vi "IMAQ FPGA Camera Link Pixel Packer U16x4.vi"(8 "Input Valid":bool, 9 "Frame Valid In":bool, 10 "Line Valid In":bool, 11 "Pixels In":u16[](array[numeric])=[0, 0, 0, 0]) -> (0 "Output Valid":bool, 1 "Frame Valid Out":bool, 2 "Line Valid Out":bool, 3 "Pixel Bus x8 Out":cluster{"Pixels":u16[], "DV":bool[]})   [LabVIEW 2020]
doc: "The Pixel Packer combines pixels from different cycles to create a Pixel Bus with 8 adjacent pixels. The DV flag in the Pixel Bus x8 Out indicates if the corresponding pixel is valid in case there are cameras with a width that is not a multiple of 8."
uses:
  <vilib>/visionFPGA/Basics/Camera Link Acquisition/Controls/IMAQ FPGA Camera Link Pixel Packer State.ctl
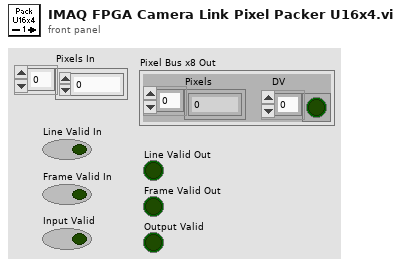
[diagram p1: front panel]
types:
  T1 = typedef "IMAQ FPGA Camera Link Pixel Packer State.ctl" = enum16{"Wait to Pack", "Pack", "Add EOL", "Check EOI"}
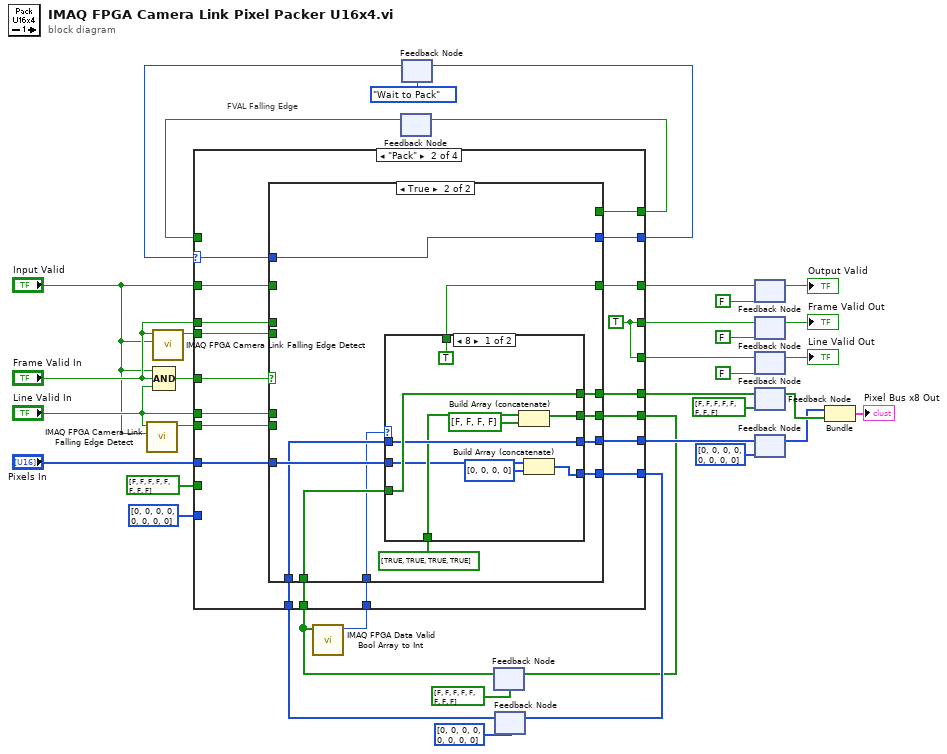
[diagram p0: block diagram]
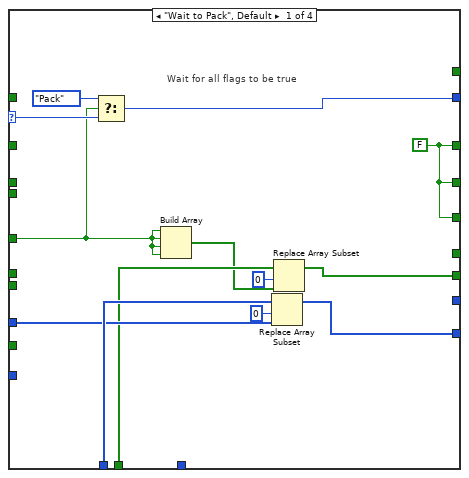
[diagram p2: hidden frame]
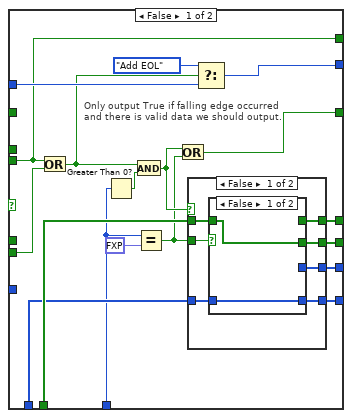
[diagram p3: hidden frame]
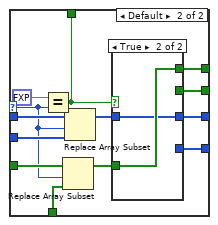
[diagram p6: hidden frame]
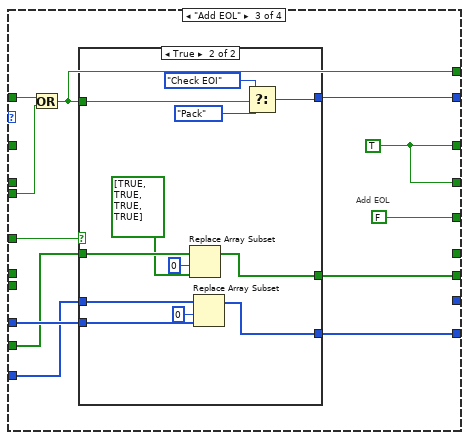
[diagram p8: hidden frame]
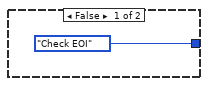
[diagram p9: hidden frame]
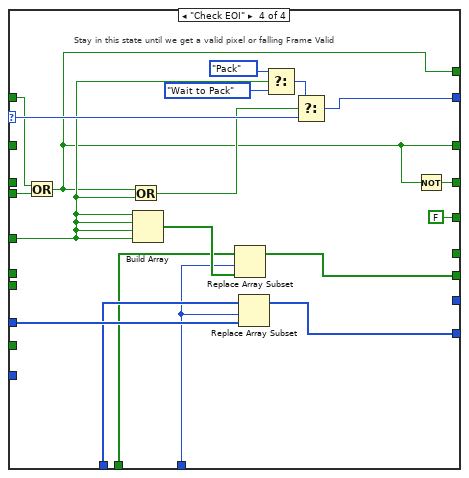
[diagram p10: hidden frame]
diagram:
  # "FVAL Falling Edge"
  n1 = call <vilib>:"IMAQ FPGA Camera Link Falling Edge Detect.vi"("Input Valid"="Input Valid", "Input"="Line Valid In") -> ("Falling Edge"=w7:bool)  [unwired: 9 in]
  n2 = call <vilib>:"IMAQ FPGA Camera Link Falling Edge Detect.vi"("Input Valid"="Input Valid", "Input"="Frame Valid In") -> ("Falling Edge"=w10:bool)  [unwired: 9 in]
  n3 = Compound Arithmetic op=AND("Input Valid", "Frame Valid In", "Line Valid In") -> (w16:bool)
  n4 = feedback #1() -> (w3:bool)  [unwired: 1 in]
  n5 = feedback #2(IMAQ_FPGA_Camera_Link_Pixel_Packer_State."Wait to Pack" ("Enum")) -> (w18:T1)
  n6 = feedback #3(bool[] [FALSE, FALSE, FALSE, FALSE, FALSE, FALSE, FALSE, FALSE]) -> (w2:bool[])
  n7 = call <vilib>:"IMAQ FPGA Data Valid Bool Array to Int.vi"("DV In"=w2) -> ("Sum DV Out"=w1:u8)  [unwired: 10 in]
  n8 = feedback #4(u16[] [0, 0, 0, 0, 0, 0, 0, 0] ("Pixels")) -> (w30:u16[])
  n9 = case shown="\"Pack\"" w18 {
    selector: w18 -> [w50 w68 _ w181]
    tunnel: w2 -> [w44 w56 _ w163]
    tunnel: w30 -> [w48 w67 _ w165]
    tunnel: [_ w64 _ _] -> w29
    tunnel: [_ w63 _ _] -> w22
    tunnel: [w38 w62 w149 w166] -> w36
    tunnel: [w38 w53 w149 w168] -> w20
    tunnel: [w38 w53 FALSE FALSE ("Frame Valid In")] -> w19
    tunnel: "Frame Valid In" -> [_ w60 _ _]
    tunnel: "Line Valid In" -> [_ w61 _ _]
    tunnel: "Input Valid" -> [_ w59 _ _]
    tunnel: w16 -> [w40 w69 w148 w172]
    tunnel: "Pixels In" -> [w46 w57 w145 w176]
    tunnel: [w45 w66 w144 w174] -> w14
    tunnel: [w42 w65 w146 w175] -> w13
    tunnel: [w41 w58 w147 w180] -> w12
    tunnel: w10 -> [_ w55 w140 w170]
    tunnel: w7 -> [_ w54 _ _]
    tunnel: u16[] [0, 0, 0, 0, 0, 0, 0, 0] ("Pixels") -> [_ _ w142 _]
    tunnel: bool[] [FALSE, FALSE, FALSE, FALSE, FALSE, FALSE, FALSE, FALSE] -> [_ _ w141 _]
    tunnel: [_ w52 w138 w166] -> w4
    tunnel: w3 -> [_ _ w139 w169]
    tunnel: w1 -> [_ w51 _ w164]
    frame "Wait to Pack", Default {
      w38 = FALSE
      # "Wait for all flags to be true"
      n10 = Select(t=IMAQ_FPGA_Camera_Link_Pixel_Packer_State."Pack", s=w40, f=w50) -> (s? t:f=w41:T1)
      n11 = Build Array(w40, w40, w40, w40) -> (w39:bool[])
      n12 = Replace Array Subset(array=w48, new element=w46, index=0) -> (w45:u16[])
      n13 = Replace Array Subset(array=w44, new element=w39, index=0) -> (w42:bool[])
    }
    frame "Pack" {
      w53 = TRUE ("Frame Valid In")
      n14 = case shown="True" w69 {
        tunnel: w68 -> [w86 w110]
        tunnel: [w84 w110] -> w58
        tunnel: w67 -> [w80 w105]
        tunnel: [w76 w103] -> w66
        tunnel: w56 -> [w81 w111]
        tunnel: [w77 w107] -> w65
        tunnel: [w78 w104] -> w64
        tunnel: [w79 w108] -> w63
        tunnel: w59 -> [_ _]
        tunnel: [w70 w109] -> w62
        tunnel: w60 -> [_ _]
        tunnel: w61 -> [_ _]
        tunnel: w55 -> [w75 _]
        tunnel: w54 -> [w87 _]
        tunnel: w51 -> [w74 w101]
        tunnel: w57 -> [_ w106]
        tunnel: [w75 _] -> w52
        frame False {
          # "Only output True if falling edge occurred and there is valid data we should output."
          n15 = Or(x=w75, y=w87) -> (x .or. y?=w82:bool)
          n16 = Greater Than 0?(x=w74) -> (x > 0?=w83:bool)
          n17 = And(x=w82, y=w83) -> (x .and. y?=w72:bool)
          n18 = Equal?(x=w74, y=fxp<+,4,4> 8.0) -> (x = y?=w71:bool)
          n19 = Or(x=w72, y=w71) -> (x .or. y?=w70:bool)
          n20 = case shown="False" w72 {
            tunnel: w81 -> [w92 w100]
            tunnel: w80 -> [w91 w99]
            tunnel: [w89 w100] -> w79
            tunnel: [w88 w99] -> w78
            tunnel: [w93 _] -> w77
            tunnel: [w90 _] -> w76
            tunnel: w71 -> [w94 _]
            frame False {
              n21 = case shown="False" w94 {
                tunnel: [w96 _] -> w93
                tunnel: w92 -> [w96 w98]
                tunnel: w91 -> [w95 w97]
                tunnel: [w95 _] -> w90
                tunnel: [_ w98] -> w89
                tunnel: [_ w97] -> w88
                frame False {
                }
                frame True {
                }
              }
            }
            frame True {
            }
          }
          n22 = Select(t=IMAQ_FPGA_Camera_Link_Pixel_Packer_State."Add EOL", s=w82, f=w86) -> (s? t:f=w84:T1)
        }
        frame True {
          n23 = case shown="8" w101 {
            selector: w101 -> [_ w121]
            tunnel: w111 -> [w119 w133]
            tunnel: [TRUE w132] -> w109
            tunnel: [w119 w130] -> w108
            tunnel: [w115 w129] -> w107
            tunnel: w106 -> [w114 w128]
            tunnel: w105 -> [w118 w127]
            tunnel: [w118 w125] -> w104
            tunnel: [w112 w124] -> w103
            tunnel: bool[] [TRUE, TRUE, TRUE, TRUE] -> [w117 w122]
            frame 8 {
              n24 = Build Array (concatenate)(w117, bool[] [FALSE, FALSE, FALSE, FALSE] ("element")) -> (w115:bool[])
              n25 = Build Array (concatenate)(w114, u16[] [0, 0, 0, 0] ("array")) -> (w112:u16[])
            }
            frame Default {
              n26 = Equal?(x=fxp<+,4,4> 4.0, y=w121) -> (x = y?=w132:bool)
              n27 = Replace Array Subset(array=w133, new element=w122, index=w121) -> (w131:bool[])
              n28 = Replace Array Subset(array=w127, new element=w128, index=w121) -> (w126:u16[])
              n29 = case shown="True" w132 {
                tunnel: w131 -> [w134 w137]
                tunnel: [_ w137] -> w130
                tunnel: [w134 _] -> w129
                tunnel: w126 -> [w135 w136]
                tunnel: [_ w136] -> w125
                tunnel: [w135 _] -> w124
                frame False {
                }
                frame True {
                }
              }
            }
          }
        }
      }
    }
    frame "Add EOL" {
      w149 = TRUE
      # "Add EOL"
      n30 = Or(x=w139, y=w140) -> (x .or. y?=w138:bool)
      n31 = case shown="True" w148 {
        tunnel: [IMAQ_FPGA_Camera_Link_Pixel_Packer_State."Check EOI" ("Enum") w151] -> w147
        tunnel: w141 -> [_ w162]
        tunnel: [_ w161] -> w146
        tunnel: w142 -> [_ w160]
        tunnel: w145 -> [_ w159]
        tunnel: [_ w157] -> w144
        tunnel: w138 -> [_ w152]
        frame False {
        }
        frame True {
          n32 = Replace Array Subset(array=w162, new element=bool[] [TRUE, TRUE, TRUE, TRUE], index=0) -> (w161:bool[])
          n33 = Replace Array Subset(array=w160, new element=w159, index=0) -> (w157:u16[])
          n34 = Select(t=IMAQ_FPGA_Camera_Link_Pixel_Packer_State."Check EOI" ("Enum"), s=w152, f=IMAQ_FPGA_Camera_Link_Pixel_Packer_State."Pack" ("Enum")) -> (s? t:f=w151:T1)
        }
      }
    }
    frame "Check EOI" {
      # "Stay in this state until we get a valid pixel or falling Frame Valid"
      n35 = Or(x=w169, y=w170) -> (x .or. y?=w166:bool)
      n36 = Or(x=w166, y=w172) -> (x .or. y?=w171:bool)
      n37 = Build Array(w172, w172, w172, w172) -> (w173:bool[])
      n38 = Replace Array Subset(array=w163, new element=w173, index=w164) -> (w175:bool[])
      n39 = Replace Array Subset(array=w165, new element=w176, index=w164) -> (w174:u16[])
      n40 = Select(t=IMAQ_FPGA_Camera_Link_Pixel_Packer_State."Pack" ("Enum"), s=w172, f=IMAQ_FPGA_Camera_Link_Pixel_Packer_State."Wait to Pack" ("Enum")) -> (s? t:f=w177:T1)
      n41 = Select(t=w177, s=w171, f=w181) -> (s? t:f=w180:T1)
      n42 = Not(x=w166) -> (.not. x?=w168:bool)
    }
  }
  n43 = feedback-in #1(w4) -> ()
  n44 = feedback-in #2(w12) -> ()
  n45 = feedback-in #3(w13) -> ()
  n46 = feedback-in #4(w14) -> ()
  n47 = feedback #5(FALSE) -> (→"Output Valid":bool)
  n48 = feedback-in #5(w36) -> ()
  n49 = feedback #6(FALSE) -> (→"Frame Valid Out":bool)
  n50 = feedback-in #6(w20) -> ()
  n51 = feedback #7(FALSE) -> (→"Line Valid Out":bool)
  n52 = feedback-in #7(w19) -> ()
  n53 = feedback #8(bool[] [FALSE, FALSE, FALSE, FALSE, FALSE, FALSE, FALSE, FALSE]) -> (w27:bool[])
  n54 = feedback-in #8(w22) -> ()
  n55 = feedback #9(u16[] [0, 0, 0, 0, 0, 0, 0, 0] ("Pixels")) -> (w26:u16[])
  n56 = feedback-in #9(w29) -> ()
  n57 = Bundle("Pixels"=w26, w27) -> (→"Pixel Bus x8 Out":cluster{"Pixels":u16[], bool[]})  [unwired: 1 in]
